vi "HallMeasurementtestv3.vi"() -> ()   [LabVIEW 2011]
panel:
  out "Array":dbl[](array[numeric])=[-0.35, -0.35, -0.35, -0.35, -0.35, -0.35, -0.35, 0.0]
  in  "# Bytes to Read":i32=200
  out "error out  9":errorcluster
  in  "Save IV Excel Report(Optional)":path
  in  "Buffer size":i32=21
  in  "Delay Between Consecutive Measurements":i32=100
  in  "Max Current Amplitude (A)":dbl=2.0 min=0.0 max=3000.0 step=0.1
  in  "Min Current Amplitude (A)":dbl=-2.0 min=-1050.0 max=1050.0 step=0.1
  in  "Number of Readings (10)":i32=10 min=2 max=1024 step=1
  in  "GPIB address Keithley":string="8"
  in  "GPIB address Agilent":string="8"
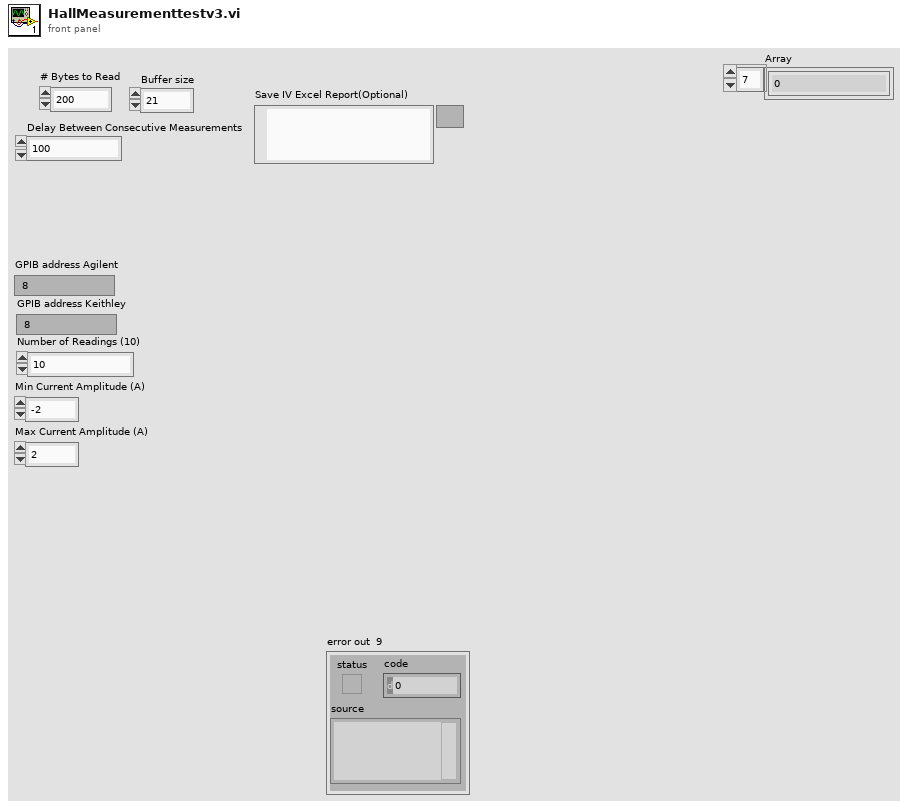
[diagram p1: front panel]
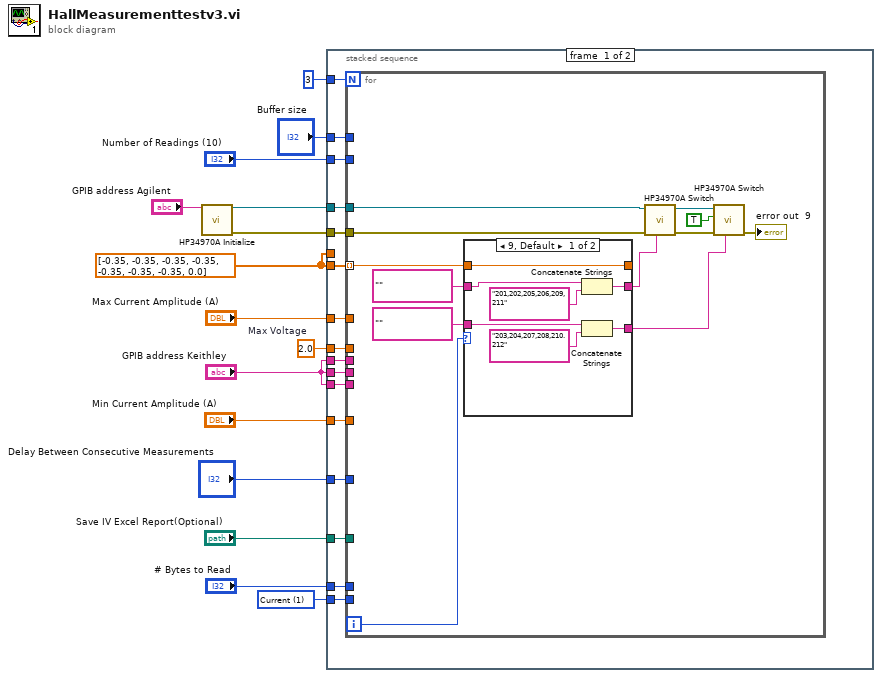
[diagram p0: block diagram]
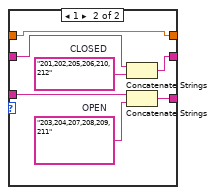
[diagram p2: hidden frame]
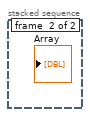
[diagram p3: hidden frame]
diagram:
  w1 = dbl[] [-0.35, -0.35, -0.35, -0.35, -0.35, -0.35, -0.35, 0.0]
  w11 = 2.0  # Max Voltage
  w8 = u16 1 items=["Volts", "Current", "Resistance"] ("Function (0: Volts)")
  n1 = call "HP34970A Initialize.vi"("VISA resource name"="GPIB address Agilent") -> ("VISA resource name out"=w14:refnum<visa-resource-name>, "error out"=w13:errorcluster)  [unwired: 13 in]
  n2 = stacked-sequence {
    tunnel: w13 -> [w31 _]
    tunnel: w14 -> [w30 _]
    tunnel: "Number of Readings (10)" -> [w27 _]
    tunnel: w11 -> [w29 _]
    tunnel: "Min Current Amplitude (A)" -> [w26 _]
    tunnel: "Max Current Amplitude (A)" -> [w28 _]
    tunnel: "GPIB address Keithley" -> [w25 _]
    tunnel: w8 -> [w24 _]
    tunnel: "Delay Between Consecutive Measurements" -> [w23 _]
    tunnel: "Buffer size" -> [w22 _]
    tunnel: "Save IV Excel Report(Optional)" -> [w21 _]
    tunnel: 3 ("Functie") -> [w20 _]
    tunnel: w1 -> [w19 _]
    tunnel: "GPIB address Keithley" -> [w18 _]
    tunnel: "GPIB address Keithley" -> [w17 _]
    tunnel: "# Bytes to Read" -> [w16 _]
    tunnel: w1 -> [_ _]
    frame #0 {
      n3 = for {
        N: w20 -> [_]
        tunnel: w31 -> [w35]
        tunnel: w30 -> [w41]
        tunnel: w29 -> [_]
        tunnel: w28 -> [_]
        tunnel: w27 -> [_]
        tunnel: w26 -> [_]
        tunnel: w25 -> [_]
        tunnel: w24 -> [_]
        tunnel: w23 -> [_]
        tunnel: w22 -> [_]
        tunnel: w21 -> [_]
        tunnel: w19 -> [w36] mode=indexing
        tunnel: w18 -> [_]
        tunnel: w17 -> [_]
        tunnel: w16 -> [_]
        i -> [w32]
        n4 = case shown="9, Default" w32 {
          tunnel: "" ("format string") -> [w47 w53]
          tunnel: "" ("format string") -> [w48 w54]
          tunnel: [w46 w52] -> w33
          tunnel: [w45 w51] -> w34
          tunnel: w36 -> [w44 w57]
          tunnel: [w44 w57] -> _
          frame 9, Default {
            n5 = Concatenate Strings(w48, "201,202,205,206,209,211" ("format string")) -> (w45:string)
            n6 = Concatenate Strings(w47, "203,204,207,208,210.212" ("format string")) -> (w46:string)
          }
          frame 1 {
            w55 = "201,202,205,206,210,212"  # CLOSED
            w56 = "203,204,207,208,209,211"  # OPEN
            n7 = Concatenate Strings(w54, w55) -> (w51:string)
            n8 = Concatenate Strings(w53, w56) -> (w52:string)
          }
        }
        n9 = call "HP34970A Switch.vi"("Channel List(empty)"=w34, "error in (no error)"=w35, "VISA resource name"=w41) -> ("error out"=w43:errorcluster, "VISA resource name out"=w40:refnum<visa-resource-name>)  [unwired: 6 in, 1 out]
        n10 = call "HP34970A Switch.vi"("Channel List(empty)"=w33, "error in (no error)"=w43, "Open/Close (F:Close)"=TRUE ("Open/Close"), "VISA resource name"=w40) -> ("error out"=→"error out  9":errorcluster)  [unwired: 5 in, 2 out]
      }
    }
    frame #1 {
    }
  }
